vi "simple PID with normalized output.vi"(6 "delta t (msec)":dbl format="%.2f", 8 "tuning parameters":T2 {"lower limit" format="%.2f"; "upper limit" format="%.2f"; "D" format="%.2f"; "I" format="%.2f"; "P" format="%.2f"}, 9 "manual input":dbl=0.5 format="%.2f", 10 "menus":T1={"setpoint type"=enum."manual", "system type"=enum."2nd ORDER"}, 11 "process variable":dbl format="%.2f") -> (0 "show slider":bool, 1 "normalized output value":dbl format="%.2f", 2 "set point":dbl format="%.2f", 3 "new process variable":dbl format="%.2f", 4 "output value":dbl format="%.2f")   [LabVIEW 2016]
doc: "This subVI emulates a control system using the create demo setpoint.vi to generate a set point value, the simple PID.vi for control, and the system type.vi to react to the PID output."
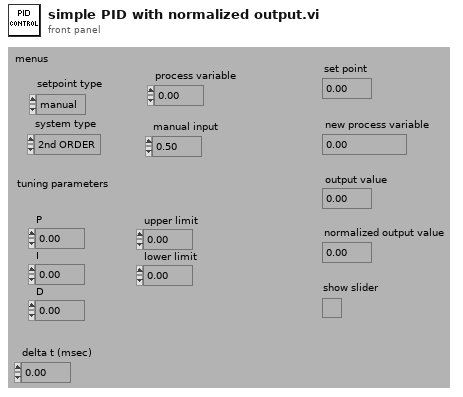
[diagram p1: front panel]
types:
  T1 = cluster{"setpoint type":enum16{"sine", "sinc", "atan", "square", "triangle", "sawtooth", "random", "manual"}, "system type":enum16{"1st ORDER", "2nd ORDER"}}
  T2 = cluster{"P":dbl, "I":dbl, "D":dbl, "upper limit":dbl, "lower limit":dbl}
  T3 = enum16{"sine", "sinc", "atan", "square", "triangle", "sawtooth", "random", "manual"}
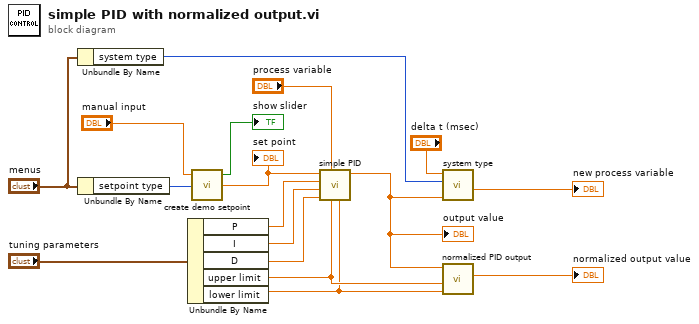
[diagram p0: block diagram]
diagram:
  n1 = Unbundle By Name("menus") -> ("system type"=w3:enum16{"1st ORDER", "2nd ORDER"})
  n2 = Unbundle By Name("menus") -> ("setpoint type"=w9:T3)
  n3 = Unbundle By Name("tuning parameters") -> ("P"=w14:dbl, "I"=w15:dbl, "D"=w16:dbl, "upper limit"=w13:dbl, "lower limit"=w12:dbl)
  n4 = call "create demo setpoint.vi"("setpoint type"=w9, "manual input"="manual input") -> ("setpoint"=w4:dbl, "show slider"=→"show slider":bool)  [unwired: 2 in]
  "set point" <- w4
  n5 = call "simple PID.vi"("lower limit"=w12, "upper limit"=w13, "process variable"="process variable", "D"=w16, "I"=w15, "P"=w14, "set point"=w4) -> ("output value"=w5:dbl)  [unwired: 4 in]
  "output value" <- w5
  n6 = call "system type.vi"("command"=w5, "system type"=w3, "delta t (msec)"="delta t (msec)") -> ("response"=→"new process variable":dbl)  [unwired: 8 in]
  n7 = call "normalized PID output.vi"("lower limit"=w12, "upper limit"=w13, "output value"=w5) -> ("normalized output value"=→"normalized output value":dbl)  [unwired: 4 in]
